vi "Write Config Changes to File.vi"(8 "error in (no error)":errorcluster, 10 "New Config":string="{}", 11 "Config File in":refnum<class "JSONConfigFile.lvclass">) -> (0 "error out":errorcluster, 2 "<JSON>Config as Written":string, 3 "Config File":refnum<class "JSONConfigFile.lvclass">, 4 "<JSON>As in file (before changes)":string)   [LabVIEW 2021, in "json.facade.lvlib" / "JSONConfigFile.lvclass"]
doc: "Write changed configuration info to the Config File. Changes are defined as differences between the input \"New Config\" and the \"Original Config\" originally Read from the file. These changes are then applied to the current Config File. \n\nNot that non-conflicting changes made to the file by another application between \"Read Config\" and \"Write Config Changes\" will not be overwritten, as only items changed by this application will be altered. This allows multiple applications or code compoenents to maintain different parameters in the same config file, without issues of race condition overwrite (as long as different apps do not alter the same item)."
uses:
  JSONConfigFile.lvclass
  JSONConfigFile.lvclass/JSONConfigFile.ctl
  jsontext/Config Files/Config File.lvclass
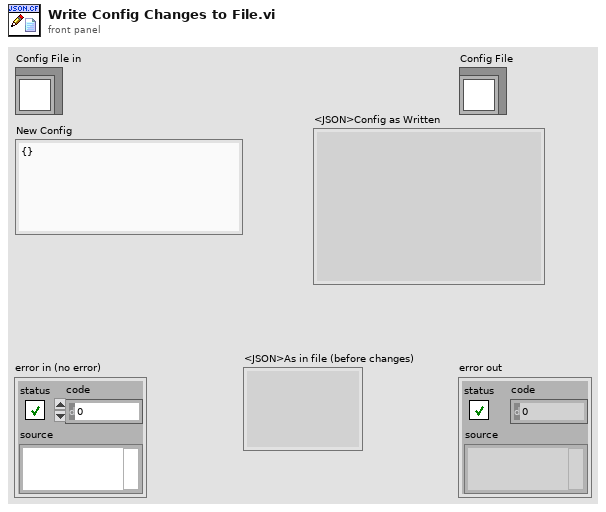
[diagram p1: front panel]
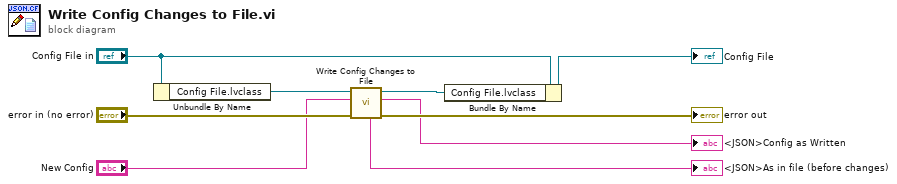
[diagram p0: block diagram]
diagram:
  n1 = Unbundle By Name("Config File in") -> ("Config File.lvclass"=w9:refnum<class "Config File.lvclass">)
  n2 = call "Write Config Changes to File.vi"("error in (no error)"="error in (no error)", "New Config"="New Config", "Config File in"=w9) -> ("error out"=→"error out":errorcluster, "<JSON>Config as Written"=→"<JSON>Config as Written":string, "Config File"=w8:refnum<class "Config File.lvclass">, "<JSON>As in file (before changes)"=→"<JSON>As in file (before changes)":string)  [unwired: 5 in]
  n3 = Bundle By Name(cluster="Config File in", "Config File.lvclass"=w8) -> (→"Config File":refnum<class "JSONConfigFile.lvclass">)
